vi "Setup--error.vi"(10 "Error":errorcluster) -> (2 "Error":errorcluster)   [LabVIEW 2020, in "jettl.lvlib" / "Error.lvlib"]
uses:
  Error.lvlib
  <vilib>/Utility/error.llb/DialogType.ctl
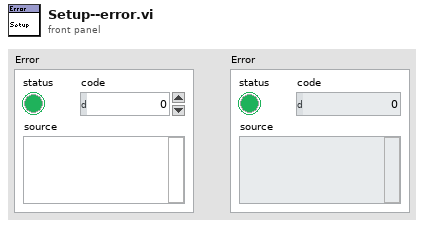
[diagram p1: front panel]
types:
  T1 = typedef "DialogType.ctl" = u16
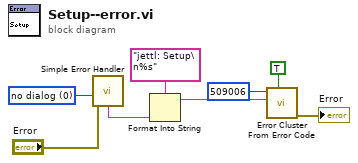
[diagram p0: block diagram]
diagram:
  w4 = T1 0 items=["no dialog", "OK message", "continue or stop message", "OK message + warnings", "continue/stop + warnings"] ("type of dialog (OK msg:1)")
  n1 = call <vilib>:"Simple Error Handler.vi"("type of dialog (OK msg:1)"=w4, "error in (no error)"="Error") -> ("message"=w3:string)  [unwired: 3 in, 4 out]
  n2 = Format Into String(format string="jettl: Setup\n%s" ("error message (\"\")"), w3) -> (resulting string=w1:string)  [unwired: 2 in, 1 out]
  n3 = call <vilib>:"Error Cluster From Error Code.vi"("show call chain? (False)"=TRUE, "error message (\"\")"=w1, "error code (0)"=509006) -> ("error out"=→"Error":errorcluster)  [unwired: 6 in]
